vi "Init Sensor Queues.vi"() -> (3 "output cluster":T1)   [LabVIEW 2013]
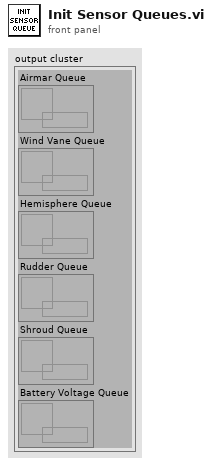
[diagram p1: front panel]
types:
  T1 = cluster{"Airmar Queue":refnum<queue>, "Wind Vane Queue":refnum<queue>, "Hemisphere Queue":refnum<queue>, "Rudder Queue":refnum<queue>, "Shroud Queue":refnum<queue>, "Battery Voltage Queue":refnum<queue>}
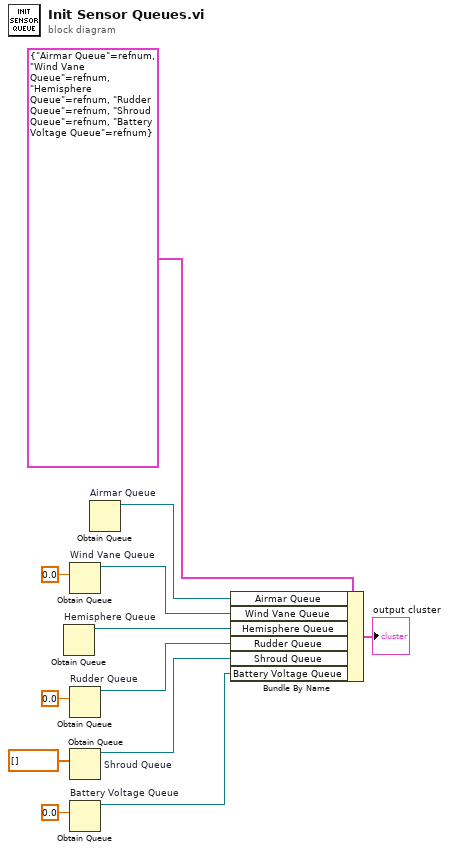
[diagram p0: block diagram]
diagram:
  n1 = Obtain Queue "Hemisphere Queue"() -> (queue out=w6:refnum<queue>)  [unwired: 5 in, 2 out]
  n2 = Obtain Queue "Wind Vane Queue"(element data type=0.0 ("x+y")) -> (queue out=w7:refnum<queue>)  [unwired: 4 in, 2 out]
  n3 = Obtain Queue "Rudder Queue"(element data type=0.0 ("x+y")) -> (queue out=w5:refnum<queue>)  [unwired: 4 in, 2 out]
  n4 = Obtain Queue "Shroud Queue"(element data type=dbl[] []) -> (queue out=w4:refnum<queue>)  [unwired: 4 in, 2 out]
  n5 = Obtain Queue "Battery Voltage Queue"(element data type=0.0 ("x+y")) -> (queue out=w1:refnum<queue>)  [unwired: 4 in, 2 out]
  n6 = Obtain Queue "Airmar Queue"() -> (queue out=w8:refnum<queue>)  [unwired: 5 in, 2 out]
  n7 = Bundle By Name(cluster=T1 {"Airmar Queue"=refnum, "Wind Vane Queue"=refnum, "Hemisphere Queue"=refnum, "Rudder Queue"=refnum, "Shroud Queue"=refnum, "Battery Voltage Queue"=refnum}, "Airmar Queue"=w8, "Wind Vane Queue"=w7, "Hemisphere Queue"=w6, "Rudder Queue"=w5, "Shroud Queue"=w4, "Battery Voltage Queue"=w1) -> (→"output cluster":T1)
